vi "Dashboard Main.vi"() -> ()   [LabVIEW 2016]
uses:
  <vilib>/Rock Robotics/Network Tables/NT Read Numeric Array.vi
  <vilib>/Rock Robotics/Network Tables/NT Write Raw.vi
panel:
  out "Camera Info":cluster{"Mbps LED":bool, "Mbps":dbl, "fps":dbl} {"fps" format="%#.1g"; "Mbps" format="%#.1g"}
  in  "Camera Settings":T1={"Frame Rate"=30, "Compression"=30, "Size"=1, "DB Camera Config"=FALSE} {"Frame Rate" scale=1.0..30.0; "Compression" scale=100.0..-1.0; "Size" items=["640x480", "320x240", "160x120"]}
  in  "TCP":refnum<k5>
  out "Robot IP":string
  in  "Dashboard Tab":enum32{"Drive", "Basic", "Custom", "Variables"}(tab)
  in  "Select Auto":string(combo)="Select Autonomous ..."
  out "NT Connection":bool
  out "MotorChart R":cluster{"Numeric":dbl, "Numeric":dbl}(graph)
  out "MotorChart L":cluster{"Numeric":dbl, "Numeric":dbl}(graph)
  out "MotorSliders R":cluster{"MotorSlide1":dbl, "MotorSlide2":dbl} {"MotorSlide2" scale=-1.0..1.0 scale format="%#_2e"; "MotorSlide1" scale=-1.0..1.0 scale format="%#_2e"}
  out "MotorSliders L":cluster{"MotorSlide1":dbl, "MotorSlide2":dbl} {"MotorSlide2" scale=-1.0..1.0 scale format="%#_2e"; "MotorSlide1" scale=-1.0..1.0 scale format="%#_2e"}
  out "JS1 Z":dbl(slide) scale=-1.0..1.0 scale format="%#_2e"
  out "JS1 Graph":cluster{"X":dbl, "Y":dbl}[](graph)
  out "JS1 Buttons":T2
  out "JS2 Z":dbl(slide) scale=-1.0..1.0 scale format="%#_2e"
  out "JS2 Graph":cluster{"X":dbl, "Y":dbl}[](graph)
  out "JS2 Buttons":T2
  out "Mode":T3(ring)=enum."Auto Disabled"
  in  "DB/String 9":string
  in  "DB/String 8":string
  in  "DB/String 7":string
  in  "DB/String 6":string
  in  "DB/String 5":string
  in  "DB/String 4":string
  in  "DB/String 3":string
  in  "DB/String 2":string
  in  "DB/String 1":string
  in  "DB/String 0":string
  in  "DB/Slider 0":dbl(slide) scale=0.0..5.0
  in  "DB/Slider 1":dbl(slide) scale=0.0..5.0
  in  "DB/Slider 2":dbl(slide) scale=0.0..5.0
  in  "DB/Slider 3":dbl(slide) scale=0.0..5.0
  out "DB/LED 3":bool
  out "DB/LED 2":bool
  out "DB/LED 1":bool
  out "DB/LED 0":bool
  in  "DB/Button 3":bool
  in  "DB/Button 2":bool
  in  "DB/Button 1":bool
  in  "DB/Button 0":bool caption="New Name"
  in  "Reset gyro?":bool
  out "Tree":string(tree)
  out "Camera Image":T4(plugin-control)
  out "Background":bool
  in  "Camera Name":string(combo)="No Camera Selection"
  # "HW"
  # "Joysticks"
  # "Drive Motors"
  # "Front"
  # "Right"
  # "Left"
  # "Back"
  # "This tab is a great place for autonomous settings and robot-specific values.\nPlace controls and indicators inside this tab and match name to\nDashboard Variables on robot. You can also delete this comment."
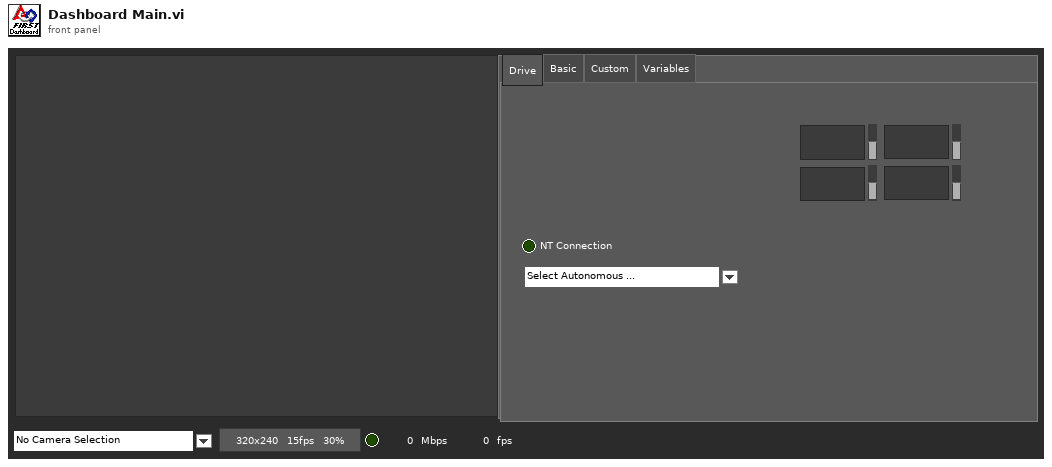
[diagram p1: front panel]
types:
  T1 = cluster{"Frame Rate":i32, "Compression":i32, "Size":u16, "DB Camera Config":bool}
  T2 = cluster{bool, bool, bool, bool, bool, bool, bool, bool, bool, bool, bool, bool}
  T3 = enum8{"Tele-Op Disabled", "Tele-Op Enabled", "Auto Disabled", "Auto Enabled", "Test Disabled", "Test Enabled", "Disconnected", "No Code", "E-Stop"}
  T4 = typedef "IMAQ Image.ctl" = refnum<image>
  T5 = enum32{"Drive", "Basic", "Custom", "Test", "Checklist", "Variables"}
  T6 = typedef "Image Type" = u32
  T7 = cluster{"Camera Image":refnum<vi>, "Dashboard Tab":refnum<vi>, "Background":refnum<vi>, "Tree":refnum<vi>, "Camera Settings":refnum<vi>, "Camera Name":refnum<vi>, "Camera Info":refnum<vi>}
  T8 = cluster{"Shift":bool, "Ctrl":bool, "Alt":bool, "Cmd":bool, "Opt":bool}
  T9 = cluster{"Error Strings":string, "Disable Counts":cluster{u16, u16}, "Rail Faults":cluster{u16, u16, u16}, "Robot IP":string, "DB Mode":u8, "Event Info":cluster{"Name":string, "Type":u8, "Number":u16, "Replay":u8}}
  T10 = cluster{"Storage":cluster{"Disk Free":u64, "RAM Block":u32, "RAM free":u32}, "CPU Utilization":cluster{"CPU % ISR":sgl, "CPU % Time Crit":sgl, "CPU % Timed Str":sgl, "CPU % High":sgl, "CPU % Above":sgl, "CPU % Normal":sgl, "CPU % Low":sgl}, "CAN":cluster{"% Bus Utilization":sgl, "Bus Off Cnt":u32, "TX_FIFO Full Cnt":u32, "Receive Error Cnt":u8, "Transmit Error Cnt":u8}, "HID":cluster{"HID Outputs":u32, "Rumble Low":u16, "Rumble High":u16}[]}
  T11 = cluster{"Status bits":cluster{"Test Mode":bool, "Autonomous":bool, "Enabled":bool, "Code Start":bool, "Brownout":bool, "Reserved 2":bool, "Reserved 3":bool, "E-Stop":bool}, "Code Trace":cluster{"Disabled":bool, "TeleOp":bool, "Auto":bool, "Test":bool}, "Controller Type":enum16{"unknown", "cRIO", "roboRio"}, "Code?":enum16{"unknown", "noCode", "code"}, "Battery V":dbl}
  T12 = cluster{"Control Bits":cluster{"TestMode":bool, "Autonomous":bool, "Enabled":bool, "FMS Present":bool, bool, bool, bool, "E-Stop":bool}, "Team Station ":u8, "Countdown":sgl, "Joystick Values":cluster{"Axes":dbl[], "Buttons":bool[], "POVs":i16[]}[]}
  T13 = cluster{"Axes":dbl[], "Buttons":bool[], "POVs":i16[]}[]
  T14 = cluster{"Axes":dbl[], "Buttons":bool[], "POVs":i16[]}
  T15 = cluster{"Buttons[0]":bool, "Buttons[1]":bool, "Buttons[2]":bool, "Buttons[3]":bool, "Buttons[4]":bool, "Buttons[5]":bool, "Buttons[6]":bool, "Buttons[7]":bool, "Buttons[8]":bool, "Buttons[9]":bool, "Buttons[10]":bool, "Buttons[11]":bool}
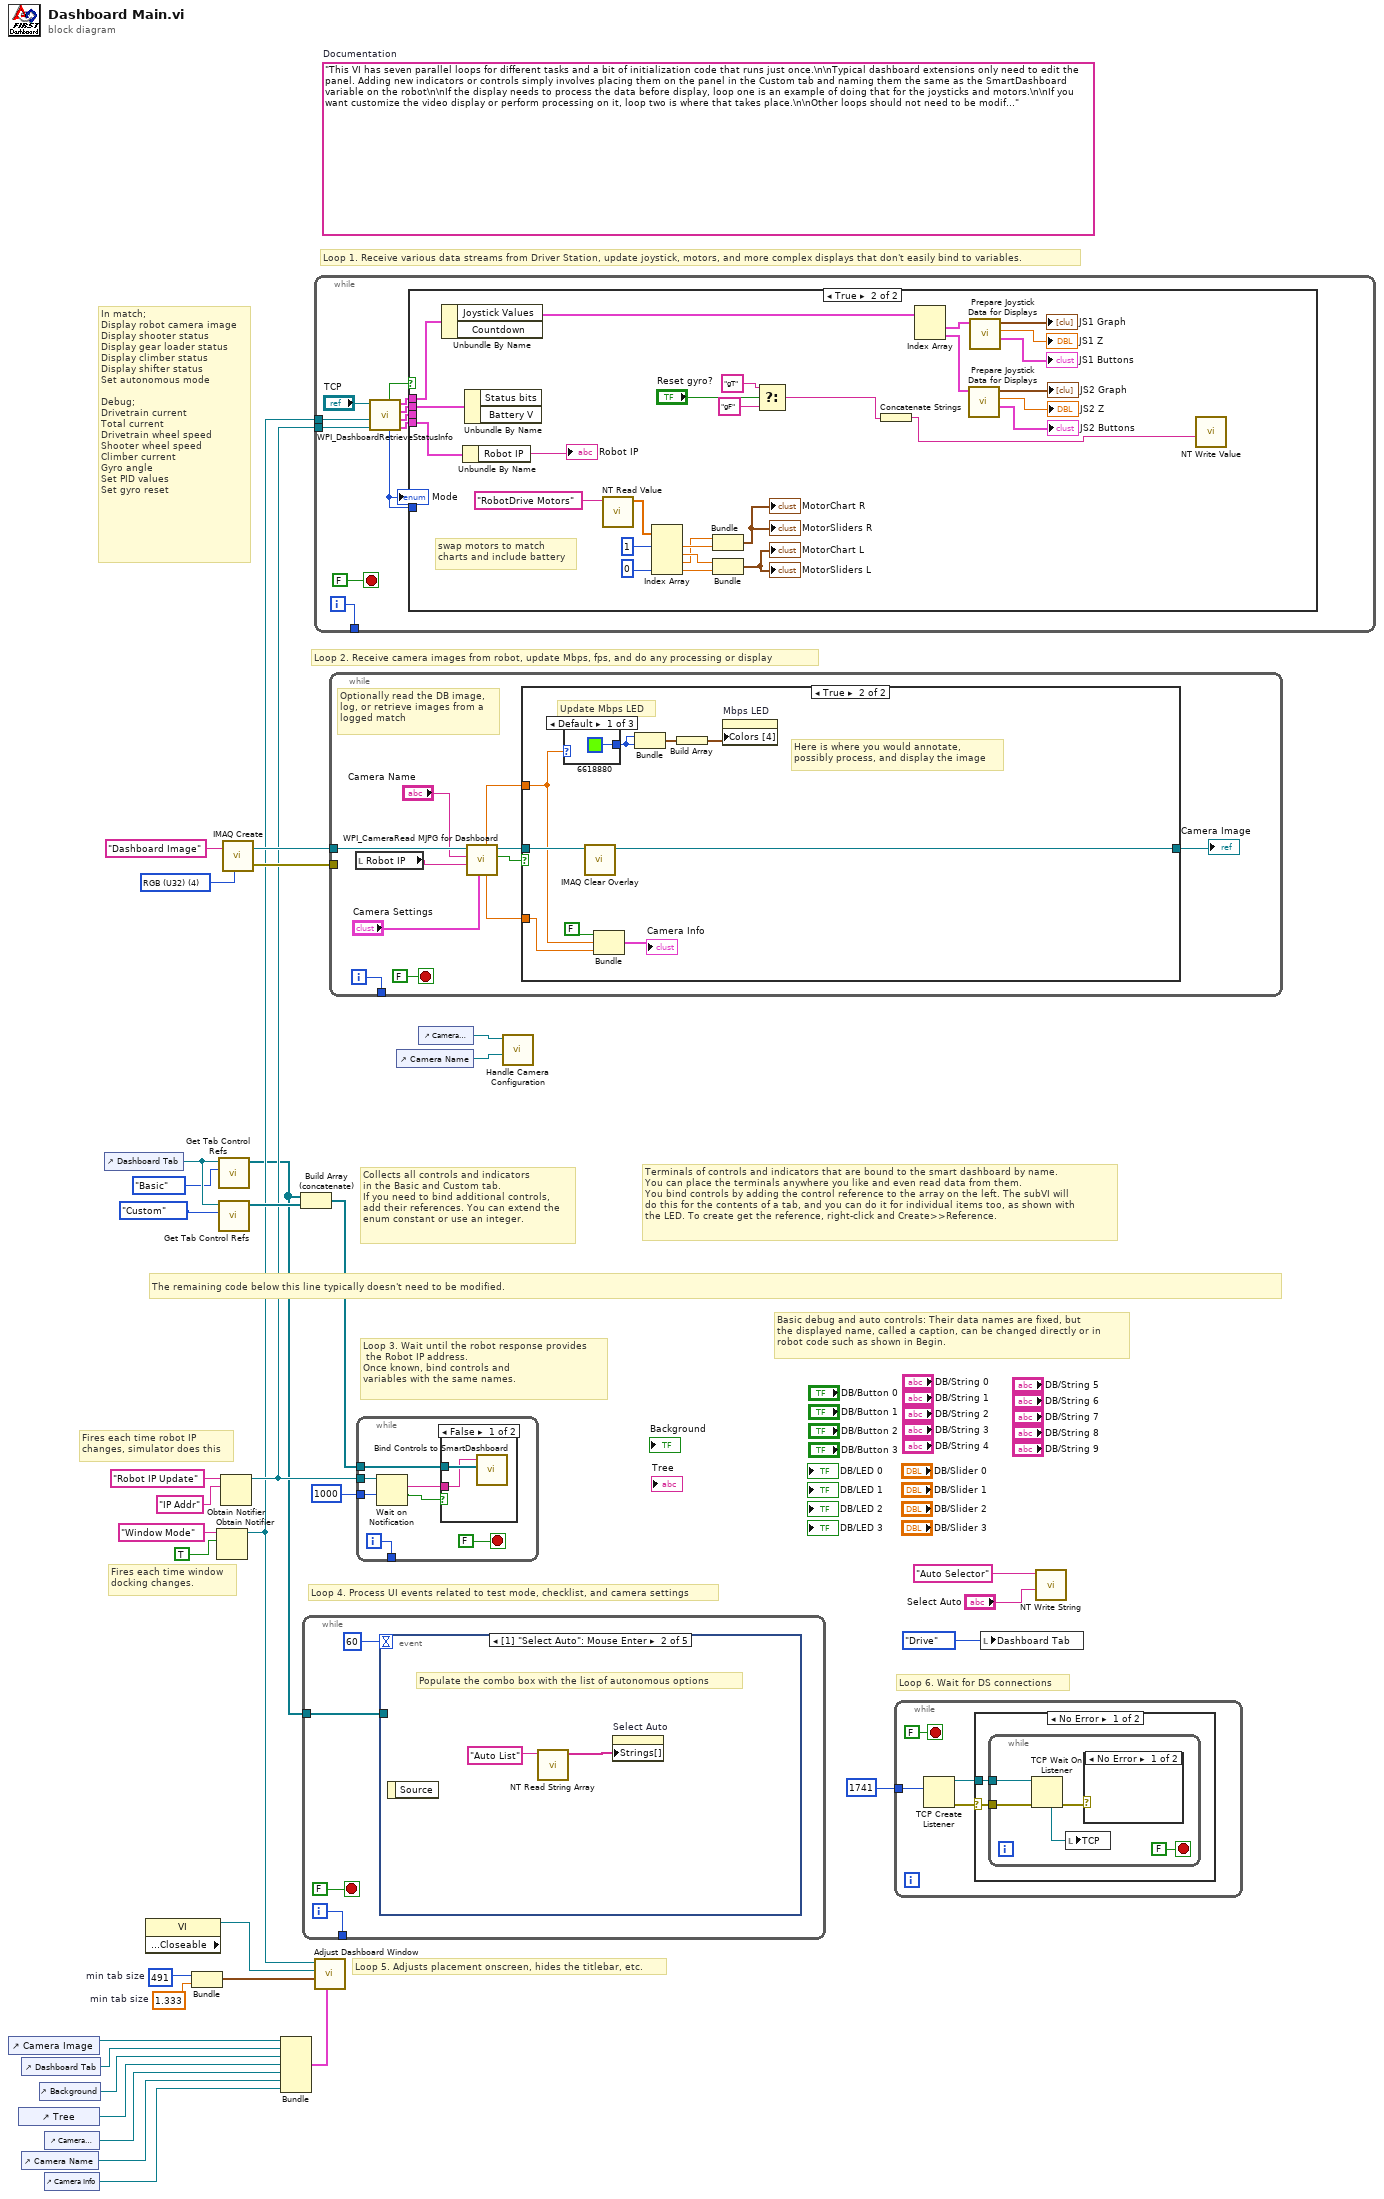
[diagram p0: block diagram]
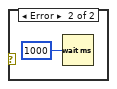
[diagram p2: hidden frame]
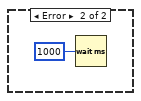
[diagram p3: hidden frame]
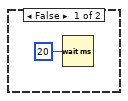
[diagram p4: hidden frame]
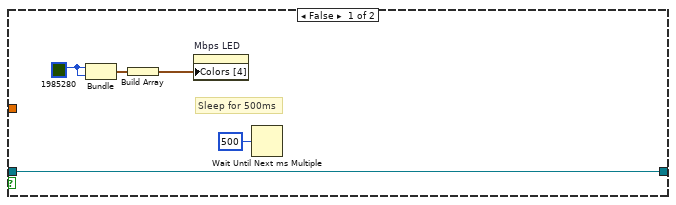
[diagram p6: hidden frame]
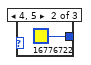
[diagram p7: hidden frame]
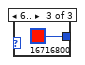
[diagram p8: hidden frame]
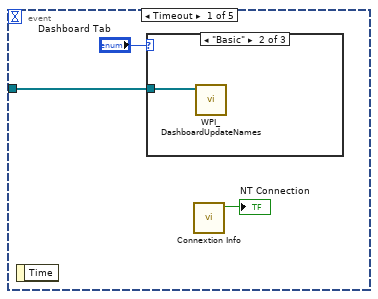
[diagram p9: hidden frame]
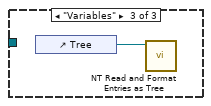
[diagram p11: hidden frame]
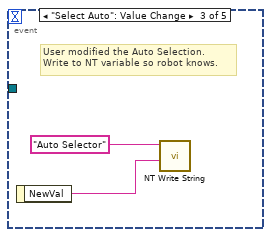
[diagram p12: hidden frame]
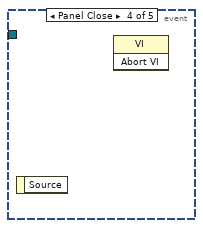
[diagram p13: hidden frame]
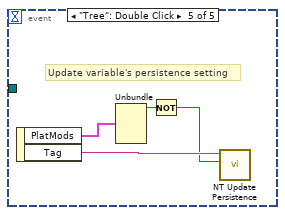
[diagram p14: hidden frame]
diagram:
  w20 = 491  # min tab size
  w19 = 1.333  # min tab size
  (unwired) "This VI has seven parallel loops for different tasks and a bit of initialization code that runs just once.\n\nTypical dashboard extensions only need to edit the panel. Adding new indicators or controls simply involves placing them on the panel in the Custom tab and naming them the same as the SmartDashboard variable on the robot\n\nIf the display needs to process the data before display, loop one is an example of doing that for the joysticks and motors.\n\nIf you want customize the video display or perform processing on it, loop two is where that takes place.\n\nOther loops should not need to be modified. They are pretty standard, and document the task they perform."  # Documentation
  w35 = T6 4 items=["Grayscale (U8)", "Grayscale (I16)", "Grayscale (SGL)", "Complex (CSG)", "RGB (U32)", "HSL (U32)", "RGB (U64)"] ("Image Type")
  # "In match;\nDisplay robot camera image\nDisplay shooter status\nDisplay gear loader status\nDisplay climber status\nDisplay shifter status\nSet autonomous mode\n\nDebug;\nDrivetrain current\nTotal current\nDrivetrain wheel speed\nShooter wheel speed\nClimber current\nGyro angle\nSet PID values\nSet gyro reset"
  # "Loop 6. Wait for DS connections"
  # "Basic debug and auto controls: Their data names are fixed, but\nthe displayed name, called a caption, can be changed directly or in\nrobot code such as shown in Begin."
  # "Fires each time robot IP\nchanges, simulator does this"
  # "Fires each time window\ndocking changes."
  # "Collects all controls and indicators\nin the Basic and Custom tab.\nIf you need to bind additional controls,\nadd their references. You can extend the\nenum constant or use an integer."
  # "The remaining code below this line typically doesn't need to be modified."
  # "Loop 4. Process UI events related to test mode, checklist, and camera settings"
  # "Terminals of controls and indicators that are bound to the smart dashboard by name.\nYou can place the terminals anywhere you like and even read data from them.\nYou bind controls by adding the control reference to the array on the left. The subVI will\ndo this for the contents of a tab, and you can do it for individual items too, as shown with\nthe LED. To create get the reference, right-click and Create>>Reference."
  # "Loop 3. Wait until the robot response provides\n the Robot IP address.\nOnce known, bind controls and\nvariables with the same names."
  # "Loop 5. Adjusts placement onscreen, hides the titlebar, etc."
  # "Loop 1. Receive various data streams from Driver Station, update joystick, motors, and more complex displays that don't easily bind to variables."
  # "Loop 2. Receive camera images from robot, update Mbps, fps, and do any processing or display"
  n1 = control-ref of="Camera Image"() -> (w22:refnum<vi>)
  n2 = control-ref of="Tree"() -> (w4:refnum<vi>)
  n3 = control-ref of="Dashboard Tab"() -> (w21:refnum<vi>)
  n4 = control-ref of="Camera Name"() -> (w2:refnum<vi>)
  n5 = control-ref of="Background"() -> (w17:refnum<vi>)
  n6 = control-ref of="Camera Settings"() -> (w3:refnum<vi>)
  n7 = control-ref of="Camera Info"() -> (w1:refnum<vi>)
  n8 = control-ref of="Dashboard Tab"() -> (w25:refnum<vi>)
  n9 = property class="VI" props=["Front Panel.Closeable"]() -> (reference out=w26:refnum<vi>)  [unwired: 2 in, 2 out]
  n10 = Bundle("min tab size"=w20, "min tab size"=w19) -> (w18:cluster{"min tab size":i32, "min tab size":dbl})  [unwired: 1 in]
  n11 = Obtain Notifier(name (unnamed)="Window Mode", notification data type=TRUE) -> (notifier out=w12:refnum<notifier>)  [unwired: 2 in, 2 out]
  n12 = call <vilib>:"Get Tab Control Refs.vi"("Page Index"=T5."Basic" ("Dashboard Tab"), "TabControl in"=w25) -> ("ControlsOnPage"=w7:refnum<vi>[])  [unwired: 9 in]
  n13 = call <vilib>:"Get Tab Control Refs.vi"("Page Index"=T5."Custom" ("Dashboard Tab"), "TabControl in"=w25) -> ("ControlsOnPage"=w24:refnum<vi>[])  [unwired: 9 in]
  n14 = Obtain Notifier(name (unnamed)="Robot IP Update", notification data type="IP Addr" ("name (unnamed)")) -> (notifier out=w13:refnum<notifier>)  [unwired: 2 in, 2 out]
  n15 = call "IMAQ Create"("Image Name"="Dashboard Image", "Image Type"=w35) -> ("New Image"=w33:T4, "error out"=w32:errorcluster)  [unwired: 2 in, 1 out]
  n16 = Bundle("Camera Image"=w22, "Dashboard Tab"=w21, "Background"=w17, "Tree"=w4, "Camera Settings"=w3, "Camera Name"=w2, "Camera Info"=w1) -> (w14:T7)  [unwired: 1 in]
  n17 = Build Array (concatenate)(w7, w24) -> (w23:refnum<vi>[])
  n18 = while {
    tunnel: [w37] -> _
    tunnel: w7 -> [w36]
    i -> [w37]
    stop <- FALSE stop-if-true
    n19 = event shown="[1] \"Select Auto\": Mouse Enter" {
      selector: _ -> [_ _ _ _ _]
      dyn-events: _ -> [_ _ _ _ _]
      timeout: u32 60 ("milliseconds to wait") -> [_ _ _ _ _]
      tunnel: w36 -> [w40 _ _ _ _]
      event Timeout {
        n20 = event-data() -> ()  [unwired: 1 in, 1 out]
        n21 = case shown="\"Basic\"" "Dashboard Tab" {
          tunnel: w40 -> [_ w43 _]
          frame "Custom", Default {
          }
          frame "Basic" {
            n22 = call <vilib>:"WPI_DashboardUpdateNames.vi"("Controls on Tab"=w43) -> ()  [unwired: 11 in]
          }
          frame "Variables" {
            n23 = control-ref of="Tree"() -> (w44:refnum<vi>)
            n24 = call <vilib>:"NT Read and Format Entries as Tree.vi"("Tree Refnum"=w44) -> ()  [unwired: 9 in, 2 out]
          }
        }
        n25 = call <vilib>:"Connextion Info.vi"() -> ("Connected"=→"NT Connection":bool)  [unwired: 10 in, 1 out]
      }
      event "Select Auto": Mouse Enter {
        # "Populate the combo box with the list of autonomous options"
        n26 = event-data() -> ()  [unwired: 1 in, 1 out]
        n27 = call <vilib>:"NT Read String Array.vi"("Name"="Auto List") -> ("String Array"=w45:string[])  [unwired: 9 in, 1 out]
        n28 = property on="Select Auto" class="CmbBox"("Strings[]"=w45) -> ()  [unwired: 2 in, 2 out]
      }
      event "Select Auto": Value Change {
        # "User modified the Auto Selection.\nWrite to NT variable so robot knows."
        n29 = event-data() -> ("NewVal"=w47:string)  [unwired: 1 in]
        n30 = call <vilib>:"NT Write String.vi"("String"=w47, "Name"="Auto Selector") -> ()  [unwired: 9 in, 1 out]
      }
      event Panel Close {
        n31 = event-data() -> ()  [unwired: 1 in, 1 out]
        n32 = invoke class="VI" method="Abort VI"() -> ()  [unwired: 3 in, 3 out]
      }
      event "Tree": Double Click {
        # "Update variable's persistence setting"
        n33 = event-data() -> ("PlatMods"=w52:T8, "Tag"=w51:string)  [unwired: 1 in]
        n34 = Unbundle(w52) -> ("Shift"=w50:bool)  [unwired: 4 out]
        n35 = Not(x=w50) -> (.not. x?=w49:bool)
        n36 = call <vilib>:"NT Update Persistence.vi"("Persistence"=w49, "Name"=w51) -> ()  [unwired: 9 in, 1 out]
      }
    }
  }
  n37 = while {
    tunnel: [w62] -> _
    tunnel: w13 -> [w56]
    tunnel: w12 -> [w53]
    i -> [w62]
    stop <- FALSE stop-if-true
    n38 = call <vilib>:"WPI_DashboardRetrieveStatusInfo.vi"("Binding Refnum"=w56, "Window Mode Notifier"=w53, "TCP Cnx"="TCP") -> ("Power and Errors"=w57:T9, "Robot Metrics"=w60:T10, "Status Info"=w61:T11, "Control Info"=w58:T12, "Robot Mode"=w55:T3, "Process?"=w59:bool)  [unwired: 3 in]
    "Mode" <- w55
    n39 = case shown="True" w59 {
      tunnel: w61 -> [_ w92]
      tunnel: w60 -> [_ _]
      tunnel: w58 -> [_ w91]
      tunnel: w57 -> [_ w90]
      tunnel: w55 -> [_ _]
      frame False {
        n40 = Wait (ms)(milliseconds to wait=u32 20) -> ()  [unwired: 1 out]
      }
      frame True {
        # "swap motors to match\ncharts and include battery"
        n41 = Unbundle By Name(w91) -> ("Joystick Values"=w81:T13)  [unwired: 1 out]
        n42 = Unbundle By Name(w90) -> ("Robot IP"=→"Robot IP":string)
        n43 = Unbundle By Name(w92) -> ()  [unwired: 2 out]
        n44 = call-poly <vilib>:"NT Read Value.vi"("Name"="RobotDrive Motors") -> ("Numeric Array"=w71:dbl[])  [unwired: 9 in, 1 out]
        n45 = Index Array(array=w71, index #1=1, index #4=0) -> (element #1=w85:dbl, element #2=w86:dbl, element #3=w84:dbl, element #4=w89:dbl)  [unwired: 2 in]
        n46 = Bundle("Numeric"=w84, "Numeric"=w85) -> (→"MotorChart R" →"MotorSliders R":cluster{"Numeric":dbl, "Numeric":dbl})  [unwired: 1 in]
        n47 = Bundle("Numeric"=w86, "Numeric"=w89) -> (→"MotorChart L" →"MotorSliders L":cluster{"Numeric":dbl, "Numeric":dbl})  [unwired: 1 in]
        n48 = Select(t="gT", s="Reset gyro?", f="gF") -> (s? t:f=w66:string)
        n49 = Concatenate Strings(w66) -> (w65:string)
        n50 = Index Array(array=w81) -> (element #1=w80:T14, element #2=w76:T14)  [unwired: 2 in]
        n51 = call "Prepare Joystick Data for Displays.vi"("Joystick Values"=w76) -> ("Buttons"=→"JS2 Buttons":T15, "Z Axis"=→"JS2 Z":dbl, "Cartesian Data"=→"JS2 Graph":cluster{"X axis":dbl, "X axis":dbl}[])  [unwired: 8 in]
        n52 = call "Prepare Joystick Data for Displays.vi"("Joystick Values"=w80) -> ("Buttons"=→"JS1 Buttons":T15, "Z Axis"=→"JS1 Z":dbl, "Cartesian Data"=→"JS1 Graph":cluster{"X axis":dbl, "X axis":dbl}[])  [unwired: 8 in]
        n53 = call-poly <vilib>:"NT Write Value.vi"("Raw"=w65) -> ()  [unwired: 10 in, 1 out]
      }
    }
  }
  n54 = call "Adjust Dashboard Window.vi"("Sizing Refnums"=w14, "Size Constraints"=w18, "VI"=w26, "WIn Mode"=w12) -> ()  [unwired: 8 in]
  n55 = while {
    tunnel: w33 -> [w101]
    tunnel: w32 -> [_]
    tunnel: [w102] -> _
    i -> [w102]
    stop <- FALSE stop-if-true
    # "Optionally read the DB image,\nlog, or retrieve images from a\nlogged match"
    n56 = local read "Robot IP"() -> (w97:string)
    n57 = call <vilib>:"WPI_CameraRead MJPG for Dashboard.vi"("Camera Settings"="Camera Settings", "Robot IP"=w97, "Camera Name"="Camera Name", "Refnum in"=w101) -> ("Active"=w99:bool, "Refnum out"=w100:T4, "FPS"=w98:dbl, "Bandwidth (Mbps)"=w96:dbl)  [unwired: 4 in]
    n58 = case shown="True" w99 {
      tunnel: w100 -> [w104 w115]
      tunnel: w96 -> [_ w112]
      tunnel: w98 -> [_ w113]
      tunnel: [w104 w109] -> w93
      frame False {
        w106 = u32 1985280 ("Color Box")
        # "Sleep for 500ms"
        n59 = Bundle("Color Box"=w106, "Color Box"=w106) -> (w107:cluster{"Color Box":u32, "Color Box":u32})  [unwired: 1 out]
        n60 = Build Array(w107) -> (w105:cluster{"Color Box":u32, "Color Box":u32}[])
        n61 = property on="Mbps LED" class="Bool (strict)"("Colors [4]"=w105) -> ()  [unwired: 2 in, 2 out]
        n62 = Wait Until Next ms Multiple(millisecond multiple=u32 500) -> ()  [unwired: 1 out]
      }
      frame True {
        # "Here is where you would annotate,\npossibly process, and display the image"
        # "Update Mbps LED"
        n63 = case shown="Default" w112 {
          tunnel: [u32 6618880 ("Color Box") u32 16776722 ("Color Box") u32 16716800 ("Color Box")] -> w116
          frame Default {
          }
          frame 4, 5 {
          }
          frame 6.. {
          }
        }
        n64 = call "IMAQ Clear Overlay"("Image"=w115) -> ("Image Out"=w109:T4)  [unwired: 2 in, 8 out]
        n65 = Bundle(FALSE, "Bandwidth (Mbps)"=w112, "FPS"=w113) -> (→"Camera Info":cluster{bool, "Bandwidth (Mbps)":dbl, "FPS":dbl})  [unwired: 1 in]
        n66 = Bundle("Color Box"=w116, "Color Box"=w116) -> (w117:cluster{"Color Box":u32, "Color Box":u32})  [unwired: 1 out]
        n67 = Build Array(w117) -> (w114:cluster{"Color Box":u32, "Color Box":u32}[])
        n68 = property on="Mbps LED" class="Bool (strict)"("Colors [4]"=w114) -> ()  [unwired: 2 in, 2 out]
      }
    }
    "Camera Image" <- w93
  }
  n69 = while {
    tunnel: w23 -> [w127]
    tunnel: w13 -> [w125]
    tunnel: [w123] -> _
    tunnel: u32 1000 ("milliseconds to wait") -> [w122]
    i -> [w123]
    stop <- FALSE stop-if-true
    n70 = Wait on Notification(notifier=w125, timeout in ms (-1)=w122) -> (notification=w124:string, timed out?=w121:bool)  [unwired: 2 in, 2 out]
    n71 = case shown="False" w121 {
      tunnel: w127 -> [w129 _]
      tunnel: w124 -> [w128 _]
      frame False {
        n72 = call <vilib>:"Bind Controls to SmartDashboard.vi"("Bound Control Refs"=w129, "Server IP Address"=w128) -> ()  [unwired: 10 in]
      }
      frame True {
      }
    }
  }
  n73 = control-ref of="Camera Name"() -> (w8:refnum<vi>)
  n74 = control-ref of="Camera Settings"() -> (w9:refnum<vi>)
  n75 = call "Handle Camera Configuration.vi"("CameraNameRef"=w8, "ClusterRef"=w9) -> ()  [unwired: 10 in]
  n76 = while {
    tunnel: u16 1741 ("timeout ms (25000)") -> [w131]
    stop <- FALSE stop-if-true
    n77 = TCP Create Listener(10:w131) -> (0:w130:errorcluster, 3:w132:refnum<k5>)  [unwired: 4 in, 1 out]
    n78 = case shown="No Error" w130 {
      selector: w130 -> [w134 _]
      tunnel: w132 -> [w135 _]
      frame No Error {
        n79 = while {
          tunnel: w135 -> [w138]
          tunnel: w134 -> [w137]
          stop <- FALSE stop-if-true
          n80 = TCP Wait On Listener(8:w137, 11:w138) -> (0:w139:errorcluster, 4:w140:refnum<k5>)  [unwired: 2 in, 3 out]
          n81 = local write "TCP"(w140) -> ()
          n82 = case shown="No Error" w139 {
            frame No Error {
            }
            frame Error {
              n83 = Wait (ms)(milliseconds to wait=u32 1000) -> ()  [unwired: 1 out]
            }
          }
        }
      }
      frame Error {
        n84 = Wait (ms)(milliseconds to wait=u32 1000) -> ()  [unwired: 1 out]
      }
    }
  }
  n85 = local write "Dashboard Tab"(enum32{"Drive", "Basic", "Custom", "Variables"}."Drive" ("Dashboard Tab")) -> ()
  n86 = call <vilib>:"NT Write String.vi"("String"="Select Auto", "Name"="Auto Selector") -> ()  [unwired: 9 in, 1 out]
